vi "set limit (子VI).vi"(8 "Temp or Field":enum16{"Field", "Temp"}(ring), 9 "limit":T1={"Field limit"=70000.0, "Field rate limit"=200.0, "Temp limit"=400.0, "Temp low limit"=2.0, "Temp rate limit "=20.0}, 10 "rate":refnum<vi>, 11 "value":refnum<vi>) -> ()   [LabVIEW 2019, in "SubVI.lvlib"]
uses:
  limit.ctl
  SubVI.lvlib
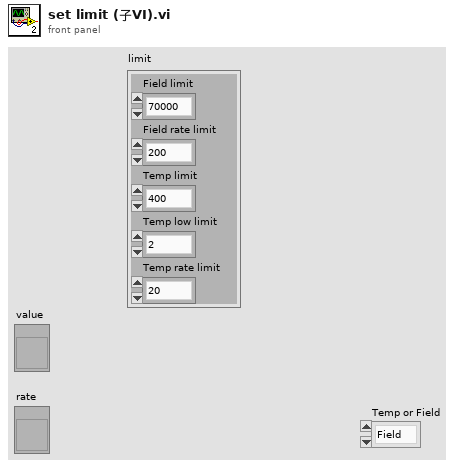
[diagram p1: front panel]
types:
  T1 = typedef "limit.ctl" = cluster{"Field limit":dbl, "Field rate limit":dbl, "Temp limit":dbl, "Temp low limit":dbl, "Temp rate limit ":dbl}
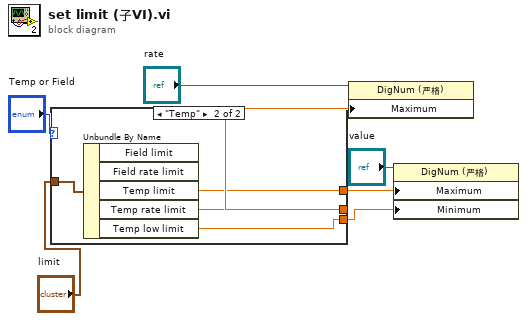
[diagram p0: block diagram]
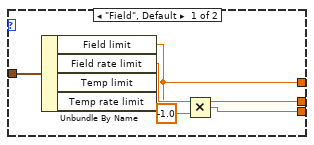
[diagram p2: hidden frame]
diagram:
  n1 = case shown="\"Temp\"" "Temp or Field" {
    tunnel: "limit" -> [w12 w16]
    tunnel: [w11 w14] -> w7
    tunnel: [w10 w15] -> w6
    tunnel: [w9 w13] -> w1
    frame "Field", Default {
      n2 = Unbundle By Name(w12) -> ("Field limit"=w10:dbl, "Field rate limit"=w11:dbl)  [unwired: 2 out]
      n3 = Multiply(x=w10, y=-1.0) -> (x*y=w9:dbl)
    }
    frame "Temp" {
      n4 = Unbundle By Name(w16) -> ("Temp limit"=w15:dbl, "Temp rate limit"=w14:dbl, "Temp low limit"=w13:dbl)  [unwired: 2 out]
    }
  }
  n5 = property on="属性节点" class="DigNum (严格)"(reference="rate", "Maximum"=w7) -> ()  [unwired: 1 in, 2 out]
  n6 = property on="属性节点" class="DigNum (严格)"(reference="value", "Maximum"=w6, "Minimum"=w1) -> ()  [unwired: 1 in, 2 out]
